vi "Initialize Sessions.vi"   [LabVIEW 2025, in "Keysight 34461A DMM Instrument.lvlib"]
doc: "Create the 34401 driver session(s) from a reservation."
uses:
  Keysight 34461A DMM Instrument.lvlib
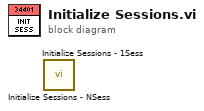
[diagram p0: block diagram]
diagram:
  n1 = call "Initialize Sessions - NSess.vi"() -> ()  [unwired: 8 in, 4 out]
  n2 = call "Initialize Sessions - 1Sess.vi"() -> ()  [unwired: 8 in, 4 out]
